vi "Sensors + UDP.vi"() -> ()   [LabVIEW 2018]
uses:
  Node 1 - States.ctl
  Shared/Globals.vi
panel:
  out "Elapsed Time (s)":dbl(slide) scale=0.0..20.0
  out "HB Signal":bool
  out "Time for HB Reading":dbl caption="Elapsed Time (s)" format="%#.2g"
  out "Current State":T1=enum."Idle"
  in  "Error Type":u16(ring) items=["General Error", "Other Node Failed", "Wifi Error"]
  out "Sensor 1":bool
  out "Sensor 2":bool
  in  "stop":bool
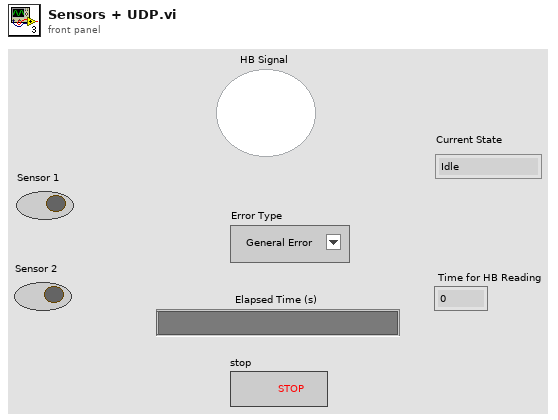
[diagram p1: front panel]
types:
  T1 = typedef "Node 1 - States.ctl" = enum16{"Initialize", "Read Sensors", "Toggle Pump", "Read HB", "Safe State", "Evaluate Error", "Log Error", "Reset Wifi", "Idle"}
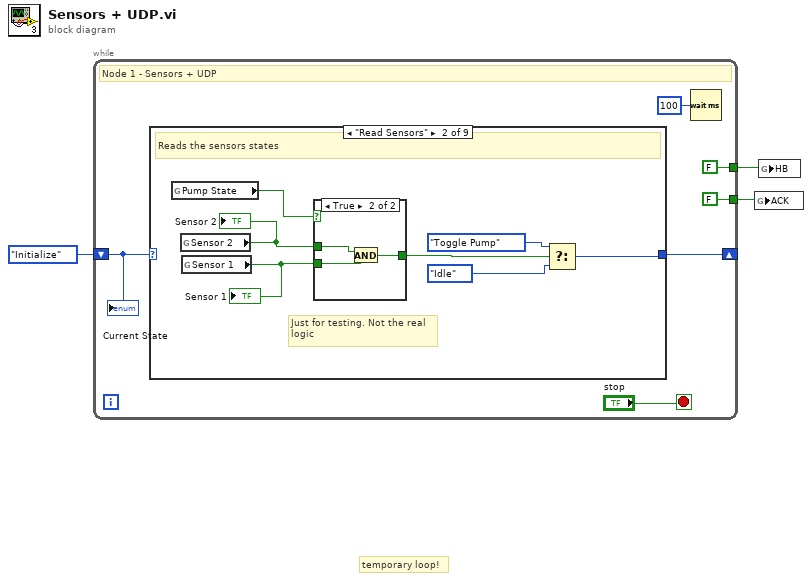
[diagram p0: block diagram]
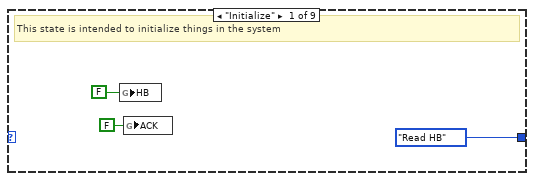
[diagram p2: hidden frame]
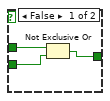
[diagram p3: hidden frame]
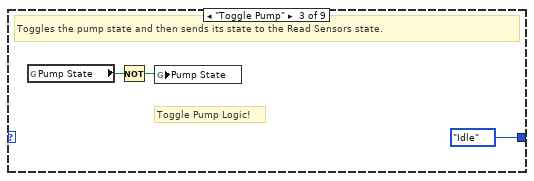
[diagram p4: hidden frame]
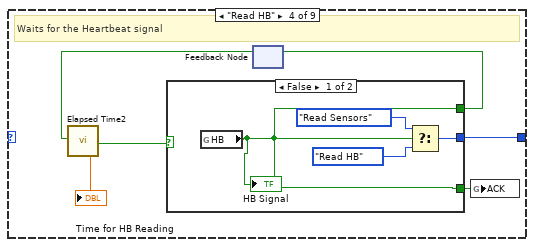
[diagram p5: hidden frame]
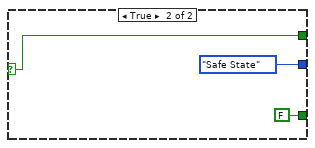
[diagram p6: hidden frame]
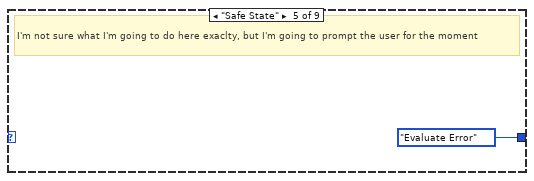
[diagram p7: hidden frame]
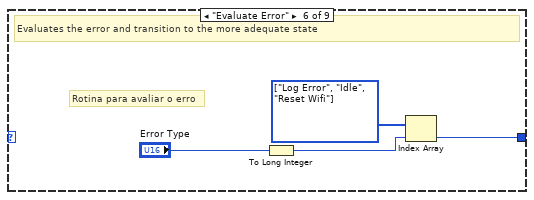
[diagram p8: hidden frame]
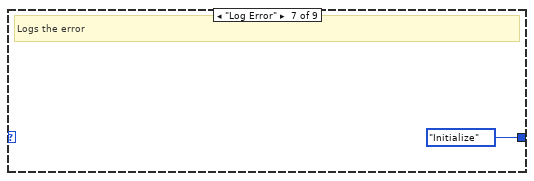
[diagram p9: hidden frame]
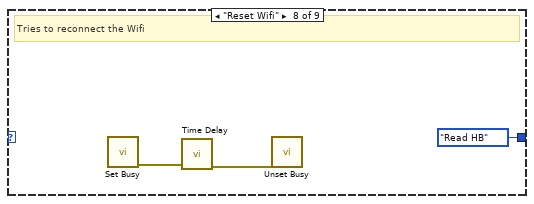
[diagram p10: hidden frame]
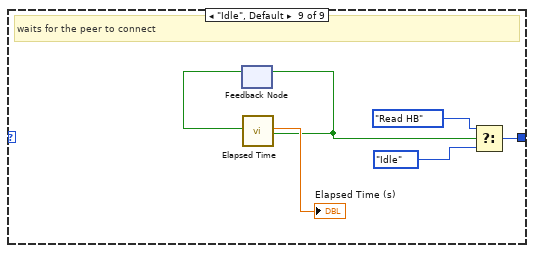
[diagram p11: hidden frame]
diagram:
  # "temporary loop!"
  n1 = while {
    shift-right: [w8] -> _
    shift-left: Node_1_-_States."Initialize" -> [w9]
    tunnel: [FALSE ("HB")] -> w2
    tunnel: [FALSE ("HB")] -> w1
    stop <- "stop" stop-if-true
    # "Node 1 - Sensors + UDP"
    n2 = case shown="\"Read Sensors\"" w9 {
      tunnel: [Node_1_-_States."Read HB" w19 Node_1_-_States."Idle" w34 Node_1_-_States."Evaluate Error" w44 Node_1_-_States."Initialize" ("Enum") Node_1_-_States."Read HB" ("Enum") w54] -> w8
      frame "Initialize" {
        # "This state is intended to initialize things in the system"
        n3 = global write "Globals.vi" "HB"(FALSE ("ACK")) -> ()
        n4 = global write "Globals.vi" "ACK"(FALSE ("ACK")) -> ()
      }
      frame "Read Sensors" {
        # "Just for testing. Not the real\nlogic"
        # "Reads the sensors states"
        n5 = global read "Globals.vi" "Pump State"() -> (w15:bool)
        n6 = global read "Globals.vi" "Sensor 2"() -> (w13:bool)
        "Sensor 2" <- w13
        n7 = global read "Globals.vi" "Sensor 1"() -> (w14:bool)
        "Sensor 1" <- w14
        n8 = case shown="True" w15 {
          tunnel: w13 -> [w21 w25]
          tunnel: w14 -> [w20 w24]
          tunnel: [w22 w23] -> w16
          frame False {
            n9 = Not Exclusive Or(1:w20, 2:w21) -> (0:w22:bool)
          }
          frame True {
            n10 = And(x=w25, y=w24) -> (x .and. y?=w23:bool)
          }
        }
        n11 = Select(t=Node_1_-_States."Toggle Pump", s=w16, f=Node_1_-_States."Idle") -> (s? t:f=w19:T1)
      }
      frame "Toggle Pump" {
        # "Toggle Pump Logic!"
        # "Toggles the pump state and then sends its state to the Read Sensors state."
        n12 = global read "Globals.vi" "Pump State"() -> (w27:bool)
        n13 = Not(x=w27) -> (.not. x?=w26:bool)
        n14 = global write "Globals.vi" "Pump State"(w26) -> ()
      }
      frame "Read HB" {
        # "Waits for the Heartbeat signal"
        n15 = feedback #1() -> (w33:bool)  [unwired: 1 in]
        n16 = call "Elapsed Time2"("Reset"=w33) -> ("Elapsed Time (s)"=→"Time for HB Reading":dbl, "Time has Elapsed"=w31:bool)  [unwired: 11 in, 6 out]
        n17 = case shown="False" w31 {
          selector: w31 -> [_ w40]
          tunnel: [w36 Node_1_-_States."Safe State"] -> w34
          tunnel: [w35 w40] -> w30
          tunnel: [w35 FALSE ("HB")] -> w29
          frame False {
            n18 = global read "Globals.vi" "HB"() -> (w35:bool)
            "HB Signal" <- w35
            n19 = Select(t=Node_1_-_States."Read Sensors", s=w35, f=Node_1_-_States."Read HB") -> (s? t:f=w36:T1)
          }
          frame True {
          }
        }
        n20 = feedback-in #1(w30) -> ()
        n21 = global write "Globals.vi" "ACK"(w29) -> ()
      }
      frame "Safe State" {
        # "I'm not sure what I'm going to do here exaclty, but I'm going to prompt the user for the moment"
      }
      frame "Evaluate Error" {
        w46 = T1[] [enum."Log Error", enum."Idle", enum."Reset Wifi"] items=["Initialize", "Read Sensors", "Toggle Pump", "Read HB", "Safe State", "Evaluate Error", "Log Error", "Reset Wifi", "Idle"]
        # "Rotina para avaliar o erro"
        # "Evaluates the error and transition to the more adequate state"
        n22 = To Long Integer(number="Error Type") -> (32bit integer=w43:i32)
        n23 = Index Array(array=w46, index=w43) -> (element=w44:T1)
      }
      frame "Log Error" {
        # "Logs the error"
      }
      frame "Reset Wifi" {
        # "Tries to reconnect the Wifi"
        n24 = call <vilib>:"Set Busy.vi"() -> ("error out"=w49:errorcluster)  [unwired: 10 in, 1 out]
        n25 = call "Time Delay"("error in (no error)"=w49) -> ("error out"=w48:errorcluster)  [unwired: 10 in]
        n26 = call <vilib>:"Unset Busy.vi"("error in (no error)"=w48) -> ()  [unwired: 10 in, 1 out]
      }
      frame "Idle", Default {
        # "waits for the peer to connect"
        n27 = feedback #2() -> (w52:bool)  [unwired: 1 in]
        n28 = call "Elapsed Time"("Reset"=w52) -> ("Elapsed Time (s)"=→"Elapsed Time (s)":dbl, "Time has Elapsed"=w51:bool)  [unwired: 11 in, 6 out]
        n29 = feedback-in #2(w51) -> ()
        n30 = Select(t=Node_1_-_States."Read HB", s=w51, f=Node_1_-_States."Idle") -> (s? t:f=w54:T1)
      }
    }
    n31 = Wait (ms)(milliseconds to wait=u32 100) -> ()  [unwired: 1 out]
    "Current State" <- w9
  }
  n32 = global write "Globals.vi" "ACK"(w2) -> ()
  n33 = global write "Globals.vi" "HB"(w1) -> ()
